vi "Initialize.vi"(8 "Error In":errorcluster, 11 "Initialization Data":variant) -> (0 "Error Out":errorcluster)   [LabVIEW 2013, in "CS++MessageLogger.lvlib"]
doc: "Initialize the central message logger."
uses:
  CS++MessageLogger.lvlib
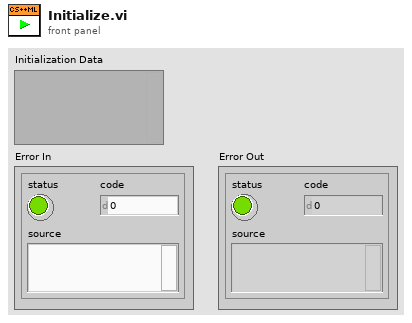
[diagram p1: front panel]
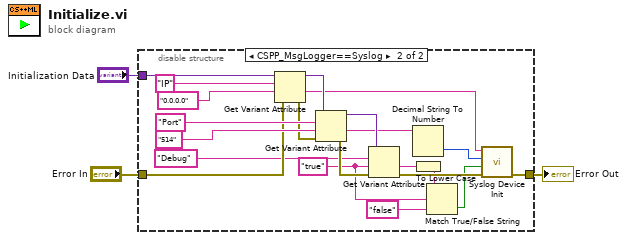
[diagram p0: block diagram]
diagram:
  n1 = disable-structure shown="CSPP_MsgLogger==Syslog" {
    disable-tunnel: "Error In" -> [w4 w14]
    disable-tunnel: [w4 w25] -> w2
    disable-tunnel: "Initialization Data" -> [_ w24]
    frame condition #0 {
    }
    frame condition #1 (active) {
      w8 = "true" ("name")
      n2 = Get Variant Attribute(Variant=w24, name="IP", default value (empty Variant)="0.0.0.0" ("name"), error in=w14) -> (duplicate Variant=w20:variant, value=w17:string, error out=w18:errorcluster)  [unwired: 1 out]
      n3 = Get Variant Attribute(Variant=w20, name="Port", default value (empty Variant)="514" ("Collector Port (514)"), error in=w18) -> (duplicate Variant=w16:variant, value=w11:string, error out=w15:errorcluster)  [unwired: 1 out]
      n4 = Get Variant Attribute(Variant=w16, name="Debug", default value (empty Variant)=w8, error in=w15) -> (value=w6:string, error out=w13:errorcluster)  [unwired: 2 out]
      n5 = Decimal String To Number(string=w11) -> (number=w10:i32)  [unwired: 2 in, 1 out]
      n6 = To Lower Case(string=w6) -> (all lower case string=w9:string)
      n7 = Match True/False String(2:"false" ("true string"), 3:w8, 4:w9) -> (0:w5:bool)  [unwired: 1 out]
      n8 = call <userlib>:"Syslog Device Init.vi"("error in (no error)"=w13, "Send debug message (T)"=w5, "Collector Port (514)"=w10, "Syslog Collector IP Address"=w17) -> ("error out"=w25:errorcluster)  [unwired: 7 in]
    }
  }
  "Error Out" <- w2
